vi "PCBdummySiCenterFinder.vi"() -> ()   [LabVIEW 2019]
uses:
  <vilib>/userDefined/High Color/IMAQdx.ctl
  Other Models/2010/Motion/AbortSingle.vi
panel:
  in  "VisibilityInCamera":enum16{"JoyStick", "ClickToMove", "AllVisible"}(ring)
  out "UsedCoordinates":string
  in  "AdjustCamera":T1={"+Y"=FALSE, "-Z"=FALSE, "Done"=FALSE, "+Z"=FALSE, "-Y"=FALSE, "-X"=FALSE, "+X"=FALSE, "MoveXYBy(mm)"=0.25, "MoveZBy(mm)"=0.1} {"MoveZBy(mm)" format="%#_13g"}
  in  "StopJoyStick":bool
  out "CameraGcode":string
  out "Image":T2(plugin-control)
  out "Deviation":dbl
  out "Output XYZU":string
  in  "PCBCorners":path=path "C:/Users/TTUHEP/Documents/LabVIEW/GantryPrograms/Configs/PCB1_4PointsA1.txt"
  in  "SiNoPatternCorners":path=path "C:/Users/TTUHEP/Documents/LabVIEW/GantryPrograms/Configs/SiDummy1Corners.txt"
  in  "Component":enum16{"SiNoPattern", "PCB"}(ring)
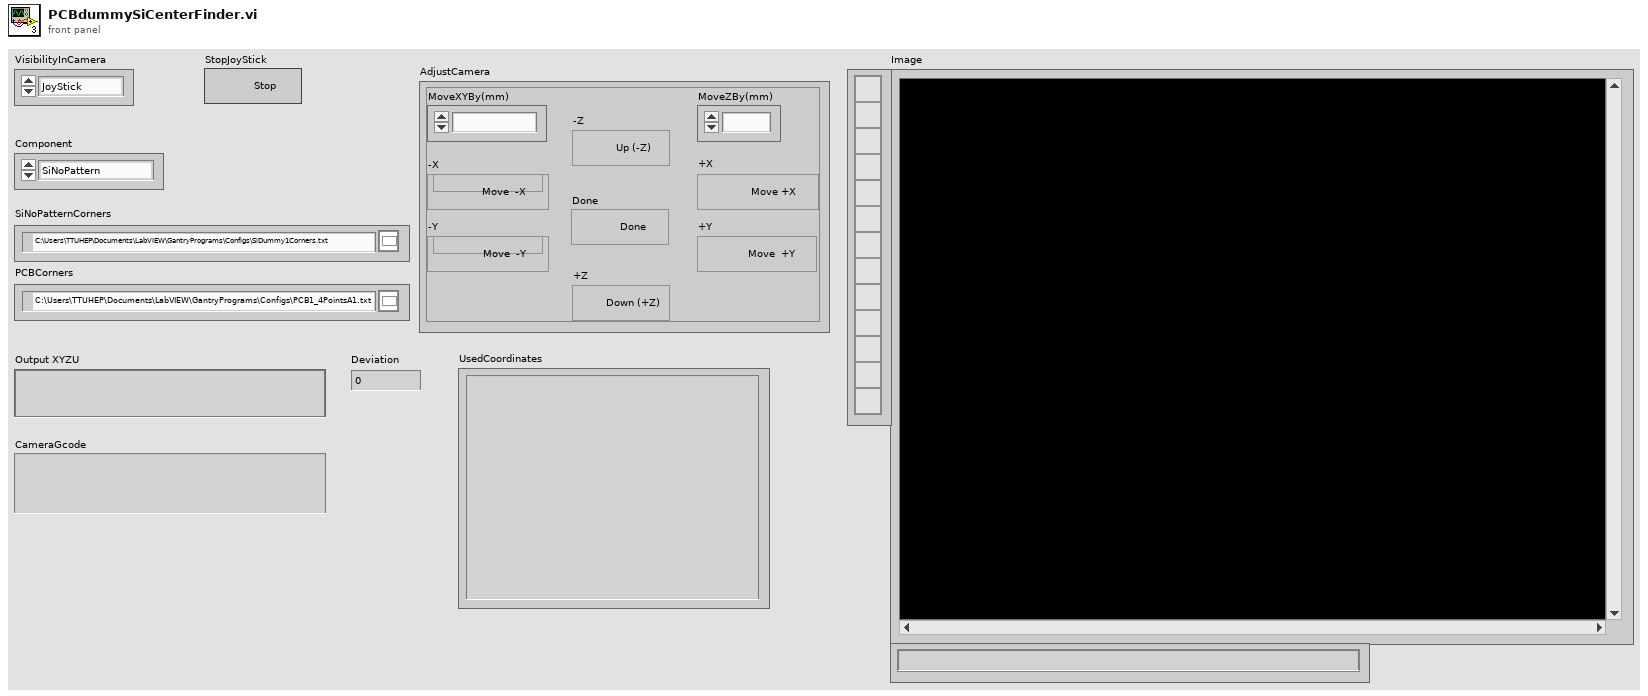
[diagram p1: front panel]
types:
  T1 = cluster{"+Y":bool, "-Z":bool, "Done":bool, "+Z":bool, "-Y":bool, "-X":bool, "+X":bool, "MoveXYBy(mm)":dbl, "MoveZBy(mm)":dbl}
  T2 = typedef "IMAQ Image.ctl" = refnum<image>
  T3 = typedef "IMAQdx.ctl" = refnum<k21>
  T4 = typedef "IMAQ Point" = cluster{"X":sgl, "Y":sgl}
  T5 = enum16{"Left Button", "Center Button", "Right Button", "Window Close"}
  T6 = enum16{"open", "replace", "create", "open or create", "replace or create", "replace or create with confirmation"}
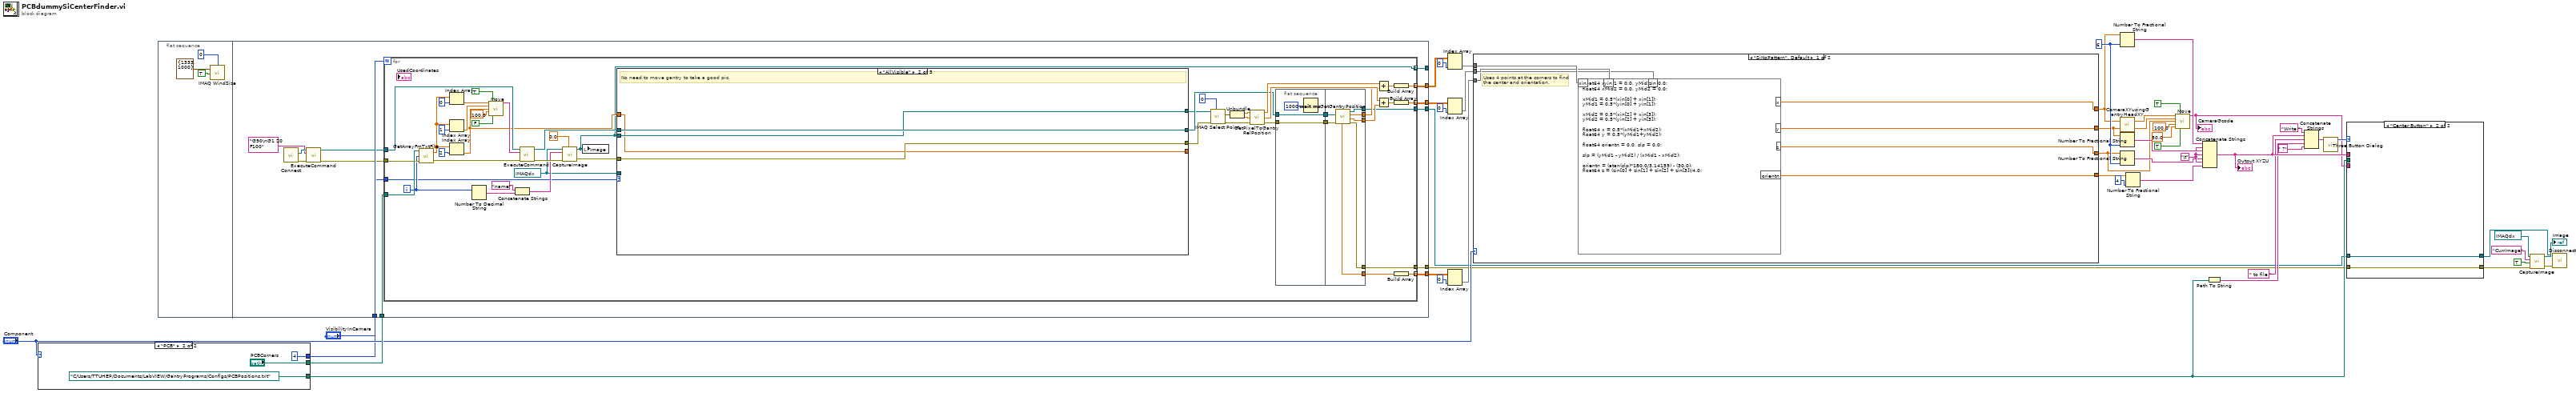
[diagram p0: block diagram]
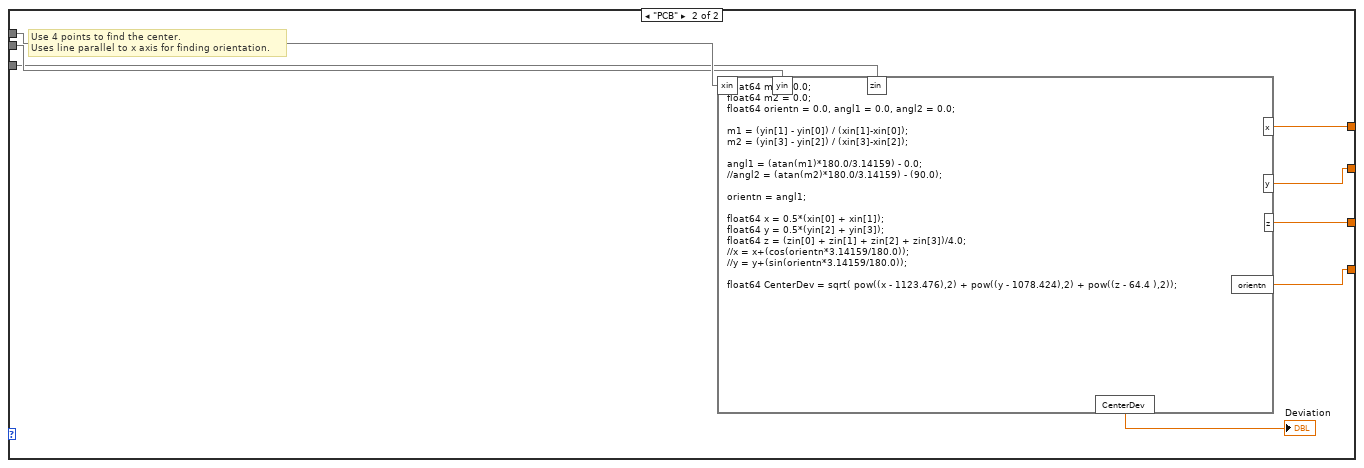
[diagram p2: hidden frame]
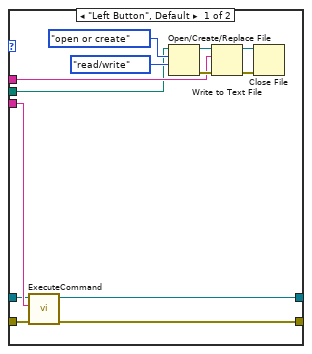
[diagram p3: hidden frame]
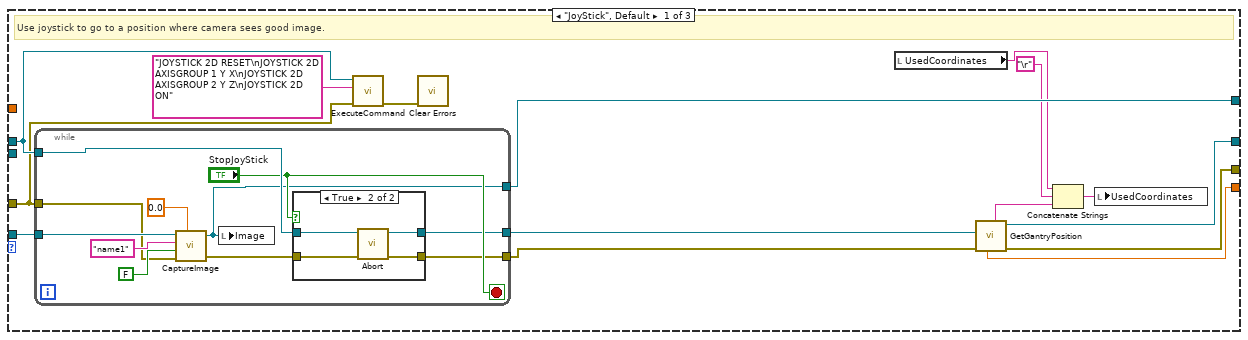
[diagram p4: hidden frame]
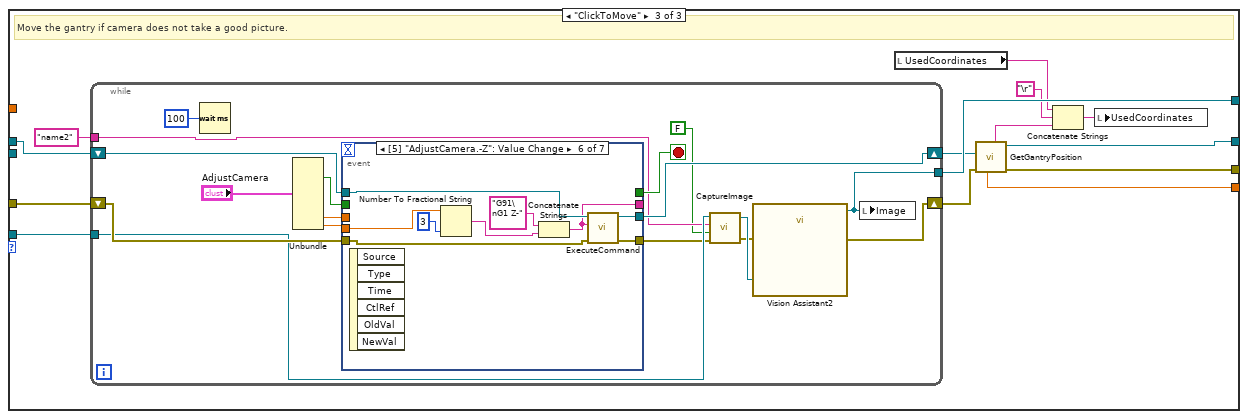
[diagram p6: hidden frame]
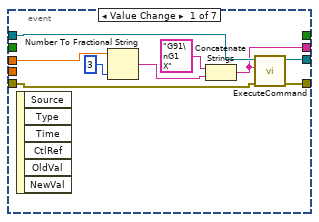
[diagram p7: hidden frame]
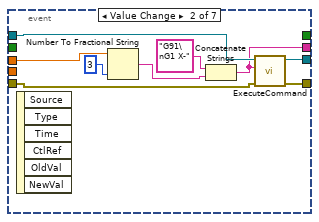
[diagram p8: hidden frame]
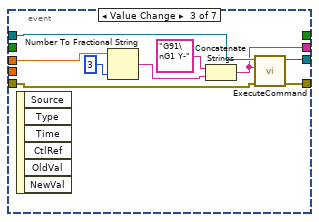
[diagram p9: hidden frame]
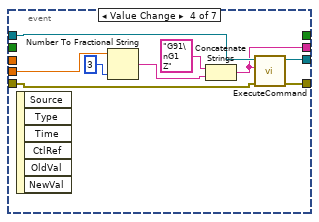
[diagram p10: hidden frame]
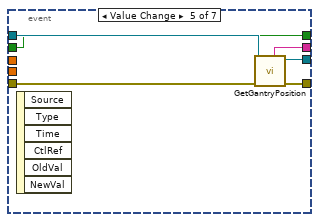
[diagram p11: hidden frame]
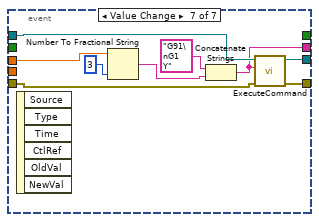
[diagram p12: hidden frame]
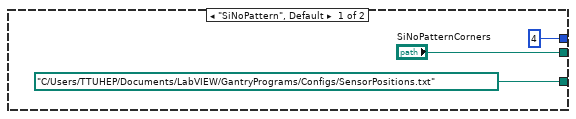
[diagram p13: hidden frame]
diagram:
  w45 = "\t"
  w42 = i16 6 ("width (-)")
  n1 = case shown="\"PCB\"" "Component" {
    tunnel: ["SiNoPatternCorners" "PCBCorners"] -> w48
    tunnel: [path "C:/Users/TTUHEP/Documents/LabVIEW/GantryPrograms/Configs/SensorPositions.txt" ("OutFile") path "C:/Users/TTUHEP/Documents/LabVIEW/GantryPrograms/Configs/PCBPositions.txt" ("OutFile")] -> w33
    tunnel: [4 4] -> w9
    frame "SiNoPattern", Default {
    }
    frame "PCB" {
    }
  }
  n2 = flat-sequence {
    tunnel: w9 -> [w71]
    tunnel: w48 -> [w70]
    tunnel: [w69] -> w7
    tunnel: [w68] -> w5
    tunnel: [w67] -> _
    tunnel: [w66] -> w31
    tunnel: [w65] -> w27
    tunnel: [w64] -> w29
    tunnel: "VisibilityInCamera" -> [w63]
    frame #0 {
      n3 = call "IMAQ WindSize"("Scrollbars? (N)"=TRUE, "Width & Height"=cluster{"Width":i32, "Height":i32} {"Width"=1333, "Height"=1000}, "Window Number"=0) -> ()  [unwired: 3 in, 3 out]
    }
    frame #1 {
      n4 = call "Connect.vi"() -> ("error out"=w62:errorcluster, "controller"=w60:refnum<k24>)  [unwired: 10 in]
      n5 = call "ExecuteCommand.vi"("error in (no error)"=w62, "Command Code"="G90\nG1 Z0 F100", "controller in"=w60) -> ("error out"=w61:errorcluster, "controller out"=w59:refnum<k24>)  [unwired: 6 in, 1 out]
      n6 = for {
        N: w71 -> [_]
        tunnel: w70 -> [w116]
        tunnel: w59 -> [w109]
        tunnel: w61 -> [w108]
        tunnel: [w88] -> w69
        tunnel: [w85] -> w68
        tunnel: [w75] -> w67 mode=indexing
        tunnel: [w102] -> w66 mode=indexing
        tunnel: [w97] -> w65 mode=indexing
        tunnel: [w96] -> w64 mode=indexing
        tunnel: w63 -> [w73]
        i -> [w106]
        w80 = T3 "cam1" ("Camera")
        n7 = call "GetArrayFmTxtFile.vi"("error in"=w108, "LineNo."=w106, "TextFile"=w116) -> ("error out"=w107:errorcluster, "Array"=w117:dbl[])
        n8 = Index Array(array=w117, index=0) -> (element=w94:dbl)
        n9 = Index Array(array=w117, index=1) -> (element=w92:dbl)
        n10 = Index Array(array=w117, index=2) -> (element=w76:dbl)
        n11 = Number To Decimal String(number=w106) -> (decimal integer string=w105:string)  [unwired: 1 in]
        n12 = call "Move.vi"("X"=w94, "Absolute"=TRUE, "Y"=w92, "Z"=w76, "SpeedXY (mm/s)"=100.0, "Move Z first"=FALSE) -> ("Position Gcode"=w110:string)  [unwired: 9 in]
        n13 = Concatenate Strings("name" ("string"), w105) -> (w103:string)
        n14 = call "ExecuteCommand.vi"("error in (no error)"=w107, "Command Code"=w110, "controller in"=w109) -> ("error out"=w112:errorcluster, "controller out"=w78:refnum<k24>)  [unwired: 6 in, 1 out]
        n15 = call "CaptureImage.vi"("Camera"=w80, "Rotate (degrees)"=sgl 0.0, "ImageName"=w103, "error in (no error)"=w112) -> ("Image"=w75:T2, "error out"=w79:errorcluster)  [unwired: 3 in]
        n16 = local write "Image"(w75) -> ()
        n17 = case shown="\"AllVisible\"" w73 {
          tunnel: w80 -> [w134 _ w169]
          tunnel: w78 -> [w132 w155 w168]
          tunnel: w79 -> [w130 w156 w167]
          tunnel: [w133 w154 w166] -> w74
          tunnel: [w128 w155 w159] -> w77
          tunnel: [w126 w156 w157] -> w72
          tunnel: w75 -> [_ w154 _]
          tunnel: [w121 w153 w158] -> _
          tunnel: w76 -> [_ w153 _]
          frame "JoyStick", Default {
            # "Use joystick to go to a position where camera sees good image."
            n18 = while {
              tunnel: w134 -> [w145]
              tunnel: [w136] -> w133
              tunnel: w132 -> [w142]
              tunnel: [w139] -> w127
              tunnel: [w138] -> w129
              tunnel: w130 -> [w137]
              stop <- "StopJoyStick" stop-if-true
              n19 = call "CaptureImage.vi"("Camera"=w145, "Rotate (degrees)"=sgl 0.0, "ImageName"="name1", "Draw50MicroCircleAtCenter"=FALSE, "error in (no error)"=w137) -> ("Image"=w136:T2, "error out"=w140:errorcluster)  [unwired: 2 in]
              n20 = local write "Image"(w136) -> ()
              n21 = case shown="True" "StopJoyStick" {
                tunnel: w142 -> [w148 w152]
                tunnel: w140 -> [w147 w151]
                tunnel: [w147 w150] -> w139
                tunnel: [w148 w149] -> w138
                frame False {
                }
                frame True {
                  n22 = call-poly "Abort.vi"("error in (no error)"=w151, "controller in"=w152) -> ("error out"=w150:errorcluster, "controller out"=w149:refnum<k24>)  [unwired: 8 in]
                }
              }
            }
            n23 = call "ExecuteCommand.vi"("error in (no error)"=w130, "Command Code"="JOYSTICK 2D RESET\nJOYSTICK 2D AXISGROUP 1 Y X\nJOYSTICK 2D AXISGROUP 2 Y Z\nJOYSTICK 2D ON", "controller in"=w132) -> ("error out"=w131:errorcluster)  [unwired: 6 in, 2 out]
            n24 = call <vilib>:"Clear Errors.vi"("error in (no error)"=w131) -> ()  [unwired: 5 in, 2 out]
            n25 = local read "UsedCoordinates"() -> (w124:string)
            n26 = call "GetGantryPosition.vi"("error in (no error)"=w127, "Controller In"=w129) -> ("error out"=w126:errorcluster, "controller out"=w128:refnum<k24>, "Position_XYZ"=w122:string, "Position Z"=w121:dbl)  [unwired: 3 in, 3 out]
            n27 = Concatenate Strings(w124, "\r", w122) -> (w125:string)
            n28 = local write "UsedCoordinates"(w125) -> ()
          }
          frame "AllVisible" {
            # "No need to move gantry to take a good pic."
          }
          frame "ClickToMove" {
            # "Move the gantry if camera does not take a good picture."
            n29 = while {
              shift-right: [w179] -> w161
              shift-left: w167 -> [w187]
              shift-right: [w185] -> w160
              shift-left: w168 -> [w186]
              tunnel: "name2" ("ImageName") -> [w181]
              tunnel: w169 -> [w182]
              tunnel: [w171] -> w166
              stop <- w184 stop-if-true
              n30 = Wait (ms)(milliseconds to wait=u32 100) -> ()  [unwired: 1 out]
              n31 = Unbundle("AdjustCamera") -> ("Done"=w175:bool, "MoveXYBy(mm)"=w173:dbl, "MoveZBy(mm)"=w174:dbl)  [unwired: 6 out]
              n32 = event shown="[5] \"AdjustCamera.-Z\": Value Change" {
                selector: _ -> [_ _ _ _ _ _ _]
                dyn-events: _ -> [_ _ _ _ _ _ _]
                timeout: _ -> [_ _ _ _ _ _ _]
                tunnel: w173 -> [w193 w197 w206 _ _ _ w239]
                tunnel: w187 -> [w192 w201 w210 w219 w228 w234 w243]
                tunnel: [w191 w200 w209 w216 w225 w233 w242] -> w180
                tunnel: w186 -> [w190 w202 w211 w220 w229 w235 w244]
                tunnel: [w189 w199 w208 w217 w227 w232 w241] -> w185
                tunnel: [w188 w198 w207 w218 w226 w231 w240] -> _
                tunnel: [_ _ _ _ w224 _ _] -> w184
                tunnel: w174 -> [_ _ _ w215 _ w230 _]
                tunnel: w175 -> [_ _ _ _ w224 _ _]
                event "AdjustCamera.+X": Value Change {
                  n33 = event-data() -> ()  [unwired: 1 in, 6 out]
                  n34 = Number To Fractional String(number=w193, precision (6)=3) -> (F-format string=w196:string)  [unwired: 2 in]
                  n35 = Concatenate Strings("G91\nG1 X", w196) -> (w188:string)
                  n36 = call "ExecuteCommand.vi"("error in (no error)"=w192, "Command Code"=w188, "controller in"=w190) -> ("error out"=w191:errorcluster, "controller out"=w189:refnum<k24>)  [unwired: 6 in, 1 out]
                }
                event "AdjustCamera.-X": Value Change {
                  n37 = event-data() -> ()  [unwired: 1 in, 6 out]
                  n38 = Number To Fractional String(number=w197, precision (6)=3) -> (F-format string=w205:string)  [unwired: 2 in]
                  n39 = Concatenate Strings("G91\nG1 X-", w205) -> (w198:string)
                  n40 = call "ExecuteCommand.vi"("error in (no error)"=w201, "Command Code"=w198, "controller in"=w202) -> ("error out"=w200:errorcluster, "controller out"=w199:refnum<k24>)  [unwired: 6 in, 1 out]
                }
                event "AdjustCamera.-Y": Value Change {
                  n41 = event-data() -> ()  [unwired: 1 in, 6 out]
                  n42 = Number To Fractional String(number=w206, precision (6)=3) -> (F-format string=w214:string)  [unwired: 2 in]
                  n43 = Concatenate Strings("G91\nG1 Y-", w214) -> (w207:string)
                  n44 = call "ExecuteCommand.vi"("error in (no error)"=w210, "Command Code"=w207, "controller in"=w211) -> ("error out"=w209:errorcluster, "controller out"=w208:refnum<k24>)  [unwired: 6 in, 1 out]
                }
                event "AdjustCamera.+Z": Value Change {
                  n45 = event-data() -> ()  [unwired: 1 in, 6 out]
                  n46 = Number To Fractional String(number=w215, precision (6)=3) -> (F-format string=w223:string)  [unwired: 2 in]
                  n47 = Concatenate Strings("G91\nG1 Z", w223) -> (w218:string)
                  n48 = call "ExecuteCommand.vi"("error in (no error)"=w219, "Command Code"=w218, "controller in"=w220) -> ("error out"=w216:errorcluster, "controller out"=w217:refnum<k24>)  [unwired: 6 in, 1 out]
                }
                event "AdjustCamera.Done": Value Change {
                  n49 = event-data() -> ()  [unwired: 1 in, 6 out]
                  n50 = call "GetGantryPosition.vi"("error in (no error)"=w228, "Controller In"=w229) -> ("error out"=w225:errorcluster, "controller out"=w227:refnum<k24>, "Position_XYZ"=w226:string)  [unwired: 3 in, 4 out]
                }
                event "AdjustCamera.-Z": Value Change {
                  n51 = event-data() -> ()  [unwired: 1 in, 6 out]
                  n52 = Number To Fractional String(number=w230, precision (6)=3) -> (F-format string=w238:string)  [unwired: 2 in]
                  n53 = Concatenate Strings("G91\nG1 Z-", w238) -> (w231:string)
                  n54 = call "ExecuteCommand.vi"("error in (no error)"=w234, "Command Code"=w231, "controller in"=w235) -> ("error out"=w233:errorcluster, "controller out"=w232:refnum<k24>)  [unwired: 6 in, 1 out]
                }
                event "AdjustCamera.+Y": Value Change {
                  n55 = event-data() -> ()  [unwired: 1 in, 6 out]
                  n56 = Number To Fractional String(number=w239, precision (6)=3) -> (F-format string=w247:string)  [unwired: 2 in]
                  n57 = Concatenate Strings("G91\nG1 Y", w247) -> (w240:string)
                  n58 = call "ExecuteCommand.vi"("error in (no error)"=w243, "Command Code"=w240, "controller in"=w244) -> ("error out"=w242:errorcluster, "controller out"=w241:refnum<k24>)  [unwired: 6 in, 1 out]
                }
              }
              n59 = call "CaptureImage.vi"("Camera"=w182, "ImageName"=w181, "Draw50MicroCircleAtCenter"=FALSE, "error in (no error)"=w180) -> ("Image"=w178:T2, "error out"=w177:errorcluster)  [unwired: 3 in]
              n60 = call "Vision Assistant2"("Image In"=w178, "error in"=w177) -> ("Image Out"=w171:T2, "error out"=w179:errorcluster)  [unwired: 24 in]
              n61 = local write "Image"(w171) -> ()
            }
            n62 = local read "UsedCoordinates"() -> (w164:string)
            n63 = call "GetGantryPosition.vi"("error in (no error)"=w161, "Controller In"=w160) -> ("error out"=w157:errorcluster, "controller out"=w159:refnum<k24>, "Position_XYZ"=w162:string, "Position Z"=w158:dbl)  [unwired: 3 in, 3 out]
            n64 = Concatenate Strings(w164, "\r", w162) -> (w165:string)
            n65 = local write "UsedCoordinates"(w165) -> ()
          }
        }
        n66 = call "IMAQ Select Point"("Window Number (0...15)"=0, "error in (no error)"=w72, "Image In"=w74) -> ("error out"=w98:errorcluster, "Point"=w101:T4)  [unwired: 5 in, 2 out]
        n67 = Unbundle(w101) -> ("X"=w100:sgl, "Y"=w99:sgl)
        n68 = call "GetPixelToGantryRelPosition.vi"("error in (no error)"=w98, "PixelY"=w99, "PixelX"=w100) -> ("error out"=w83:errorcluster, "YmmRelGH"=w91:dbl, "XmmRelGH"=w95:dbl)
        n69 = flat-sequence {
          tunnel: w83 -> [w249]
          tunnel: [w249] -> w82
          tunnel: w77 -> [w248]
          tunnel: [w248] -> w81
          tunnel: [w257] -> w88
          tunnel: [w256] -> w87
          tunnel: [w255] -> w86
          tunnel: [w254] -> w85
          tunnel: [w253] -> w84
          tunnel: w82 -> [w252]
          tunnel: w81 -> [w251]
          frame #0 {
            n70 = Wait (ms)(milliseconds to wait=u32 1000) -> ()  [unwired: 1 out]
          }
          frame #1 {
            n71 = call "GetGantryPosition.vi"("error in (no error)"=w252, "Controller In"=w251) -> ("error out"=w257:errorcluster, "Position Y"=w256:dbl, "Position X"=w255:dbl, "controller out"=w254:refnum<k24>, "Position Z"=w253:dbl)  [unwired: 3 in, 2 out]
          }
        }
        n72 = Add(x=w95, y=w86) -> (x+y=w93:dbl)
        n73 = Add(x=w91, y=w87) -> (x+y=w90:dbl)
        n74 = Build Array(w93) -> (w96:dbl[])
        n75 = Build Array(w90) -> (w97:dbl[])
        n76 = Build Array(w84) -> (w102:dbl[])
      }
    }
  }
  n77 = Index Array(array=w29, index (col)=0 ("disabled index (col)")) -> (element=w26:dbl[])  [unwired: 1 in]
  n78 = Index Array(array=w27, index (col)=0 ("disabled index (col)")) -> (element=w25:dbl[])  [unwired: 1 in]
  n79 = Index Array(array=w31, index (col)=0 ("disabled index (col)")) -> (element=w24:dbl[])  [unwired: 1 in]
  n80 = case shown="\"SiNoPattern\", Default" "Component" {
    tunnel: w26 -> [w264 w272]
    tunnel: w25 -> [w263 w271]
    tunnel: w24 -> [w262 w270]
    tunnel: [w261 w269] -> w23
    tunnel: [w260 w268] -> w14
    tunnel: [w259 w267] -> w13
    tunnel: [w258 w266] -> w10
    frame "SiNoPattern", Default {
      # "Uses 4 points at the corners to find\nthe center and orientation."
      n81 = formula code="float64 xMid1 = 0.0, yMid1 = 0.0;\nfloat64 xMid2 = 0.0, yMid2 = 0.0;\n\nxMid1 = 0.5*(xin[0] + xin[1]);\nyMid1 = 0.5*(yin[0] + yin[1]);\n\nxMid2 = 0.5*(xin[2] + xin[3]);\nyMid2 = 0.5*(yin[2] + yin[3]);\n\nfloat64 x = 0.5*(xMid1+xMid2);\nfloat64 y = 0.5*(yMid1+yMid2);\n\nfloat64 orientn = 0.0, slp = 0.0;\n\nslp = (yMid1 - yMid2) / (xMid1 - xMid2);\n\norientn = (atan(slp)*180.0/3.14159) - (30.0);\nfloat64 z = (zin[0] + zin[1] + zin[2] + zin[3])/4.0;"("xin"=w264, "yin"=w263, "zin"=w262) -> ("orientn"=w261:dbl, "x"=w260:dbl, "y"=w259:dbl, "z"=w258:dbl)
    }
    frame "PCB" {
      # "Use 4 points to find the center.\nUses line parallel to x axis for finding orientation."
      n82 = formula code="float64 m1 = 0.0;\nfloat64 m2 = 0.0;\nfloat64 orientn = 0.0, angl1 = 0.0, angl2 = 0.0;\n\nm1 = (yin[1] - yin[0]) / (xin[1]-xin[0]);\nm2 = (yin[3] - yin[2]) / (xin[3]-xin[2]);\n\nangl1 = (atan(m1)*180.0/3.14159) - 0.0;\n//angl2 = (atan(m2)*180.0/3.14159) - (90.0);\n\norientn = angl1;\n\nfloat64 x = 0.5*(xin[0] + xin[1]);\nfloat64 y = 0.5*(yin[2] + yin[3]);\nfloat64 z = (zin[0] + zin[1] + zin[2] + zin[3])/4.0;\n//x = x+(cos(orientn*3.14159/180.0));\n//y = y+(sin(orientn*3.14159/180.0));\n\nfloat64 CenterDev = sqrt( pow((x - 1123.476),2) + pow((y - 1078.424),2) + pow((z - 64.4 ),2));"("xin"=w272, "yin"=w271, "zin"=w270) -> ("orientn"=w269:dbl, "x"=w268:dbl, "y"=w267:dbl, "z"=w266:dbl, "CenterDev"=→"Deviation":dbl)
    }
  }
  n83 = Number To Fractional String(number=w14, precision (6)=w42) -> (F-format string=w47:string)  [unwired: 2 in]
  n84 = call "CameraXYusingGantryHeadXY.vi"("GantryY"=w13, "GantryX"=w14) -> ("CamY"=w11:dbl, "CamX"=w12:dbl)
  n85 = Number To Fractional String(number=w13, precision (6)=w42) -> (F-format string=w46:string)  [unwired: 2 in]
  n86 = Number To Fractional String(number=w10, precision (6)=w42) -> (F-format string=w41:string)  [unwired: 2 in]
  n87 = Number To Fractional String(number=w23, precision (6)=i16 4 ("width (-)")) -> (F-format string=w43:string)  [unwired: 2 in]
  n88 = call "Move.vi"("X"=w12, "Absolute"=TRUE, "Y"=w11, "Z"=w10, "SpeedXY (mm/s)"=100.0, "SpeedZ (mm/s)"=50.0, "Move Z first"=TRUE) -> ("Position Gcode"=w6:string)  [unwired: 8 in]
  "CameraGcode" <- w6
  n89 = Concatenate Strings(w47, w45, w46, w45, w41, w45, w43) -> (w39:string)
  "Output XYZU" <- w39
  n90 = Path To String(path=w33) -> (string=w37:string)
  n91 = Concatenate Strings("Write ", w39, " to file ", w37, " ?" ("string")) -> (w35:string)
  n92 = call <vilib>:"Three Button Dialog.vi"("message"=w35) -> ("Which Button?"=w34:T5)  [unwired: 10 in]
  n93 = case shown="\"Center Button\"" w34 {
    tunnel: w39 -> [w279 _]
    tunnel: w33 -> [w278 _]
    tunnel: w7 -> [w277 w287]
    tunnel: w6 -> [w276 _]
    tunnel: w5 -> [w275 w286]
    tunnel: [w274 w287] -> w4
    tunnel: [w273 w286] -> w3
    frame "Left Button", Default {
      n94 = call "ExecuteCommand.vi"("error in (no error)"=w277, "Command Code"=w276, "controller in"=w275) -> ("error out"=w274:errorcluster, "controller out"=w273:refnum<k24>)  [unwired: 6 in, 1 out]
      n95 = Open/Create/Replace File(file path (use dialog)=w278, operation (0:open)=T6."open or create", access (0:read/write)=enum16{"read/write", "read-only", "write-only"}."read/write") -> (refnum out=w285:refnum<file>, error out=w282:errorcluster)  [unwired: 3 in, 1 out]
      n96 = Write to Text File(file (use dialog)=w285, text=w279, error in=w282) -> (refnum out=w280:refnum<file>, error out=w281:errorcluster)  [unwired: 1 in, 1 out]
      n97 = Close File(refnum=w280, error in=w281) -> ()  [unwired: 2 out]
    }
    frame "Center Button" {
    }
  }
  n98 = call "CaptureImage.vi"("Camera"=T3 "cam1", "ImageName"="CurrImage", "Draw50MicroCircleAtCenter"=TRUE, "error in (no error)"=w4) -> ("Image"=→"Image":T2, "error out"=w17:errorcluster)  [unwired: 3 in]
  n99 = call "Disconnect.vi"("error in (no error)"=w17, "controller"=w3) -> ()  [unwired: 9 in, 1 out]
